vi "CIMAQ_GetGaussianKernel.vi"(8 "error in (no error)":errorcluster, 10 "s":dbl format="%#_13g", 11 "Size":i32=9) -> (0 "error out":errorcluster, 3 "Kernel":u8[][](array[numeric]))   [LabVIEW 2017]
uses:
  <vilib>/Analysis/baseanly.llb/Real Outer Product.vi
  <vilib>/Analysis/NI_AALBase.lvlib
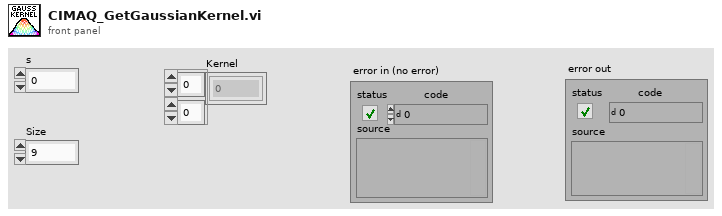
[diagram p1: front panel]
types:
  T1 = typedef "NI_Matrix.lvlib/RealMatrix.ctl" = dbl[][]
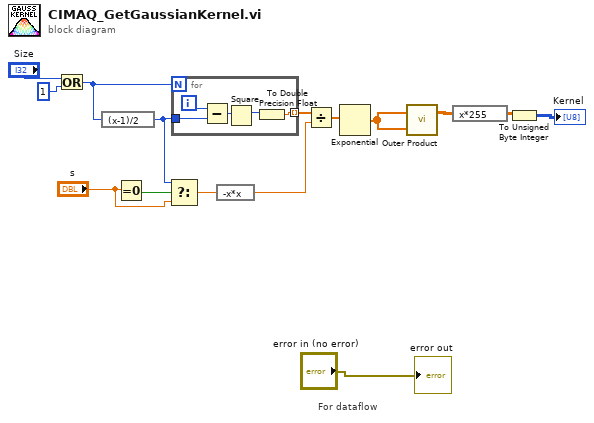
[diagram p0: block diagram]
diagram:
  # "For dataflow"
  n1 = Or(x="Size", y=1) -> (x .or. y?=w6:i32)
  n2 = expression code="(x-1)/2"(w6) -> (w8:i32)
  n3 = Equal To 0?(x="s") -> (x = 0?=w9:bool)
  n4 = Select(t=w8, s=w9, f="s") -> (s? t:f=w11:dbl)
  n5 = for {
    N: w6 -> [_]
    tunnel: w8 -> [w20]
    tunnel: [w16] -> w15 mode=indexing
    i -> [w19]
    n6 = Subtract(x=w19, y=w20) -> (x-y=w18:i32)
    n7 = Square(x=w18) -> (x^2=w17:i32)
    n8 = To Double Precision Float(number=w17) -> (double precision float=w16:dbl)
  }
  n9 = expression code="-x*x"(w11) -> (w12:dbl)
  n10 = Divide(x=w15, y=w12) -> (x/y=w14:dbl[])
  n11 = Exponential(1:w14) -> (0:w13:dbl[])
  n12 = call-poly <vilib>:"Outer Product.vi"("Y Vector"=w13, "X Vector"=w13) -> ("Outer Product"=w3:T1)  [unwired: 1 out]
  n13 = expression code="x*255"(w3) -> (w4:T1)
  n14 = To Unsigned Byte Integer(number=w4) -> (unsigned 8bit integer=→"Kernel":u8[][])
  "error out" <- "error in (no error)"
